vi "colorScatterRandomGenerator.vi"(8 "error in":errorcluster, 11 "Control in":refnum<vi>) -> (0 "error out":errorcluster)   [LabVIEW 2023]
uses:
  <vilib>/Math Plots/3D Math Plots/3D Scatter/3D Scatter XCtrl/3D Scatter.xctl
  <vilib>/Math Plots/3D Math Plots/3D Plot/3D Plot/Typedef/Color Ramp Cluster.ctl
  <vilib>/Math Plots/3D Math Plots/3D Plot/3D Plot/Typedef/Sprite Type.ctl
  <vilib>/Math Plots/3D Math Plots/3D Plot/3D Plot/3D Plot.lvclass
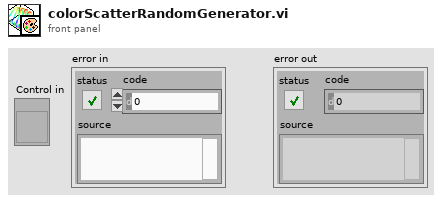
[diagram p1: front panel]
types:
  T1 = typedef "3D Plot.lvclass/Sprite Type.ctl" = enum16{"None", "Empty Square", "Solid Square", "Empty Diamond", "Solid Diamond", "Empty Circle", "Solid Circle", "Asterisk", "Bold X", "Wireframe Sphere", "Solid Sphere", "Wireframe Cube", "Solid Cube"}
  T2 = enum16{"None", "Shaded", "Color spectrum", "Grey scale", "Custom"}
  T3 = typedef "3D Plot.lvclass/Color Ramp Cluster.ctl" = cluster{"Color Ramp Style":enum16{"None", "Shaded", "Color spectrum", "Grey scale", "Custom"}, "Color Ramp Array":u32[], "Color Ramp Index":i32[], "Interpolate?":bool, "Logarithm?":bool}
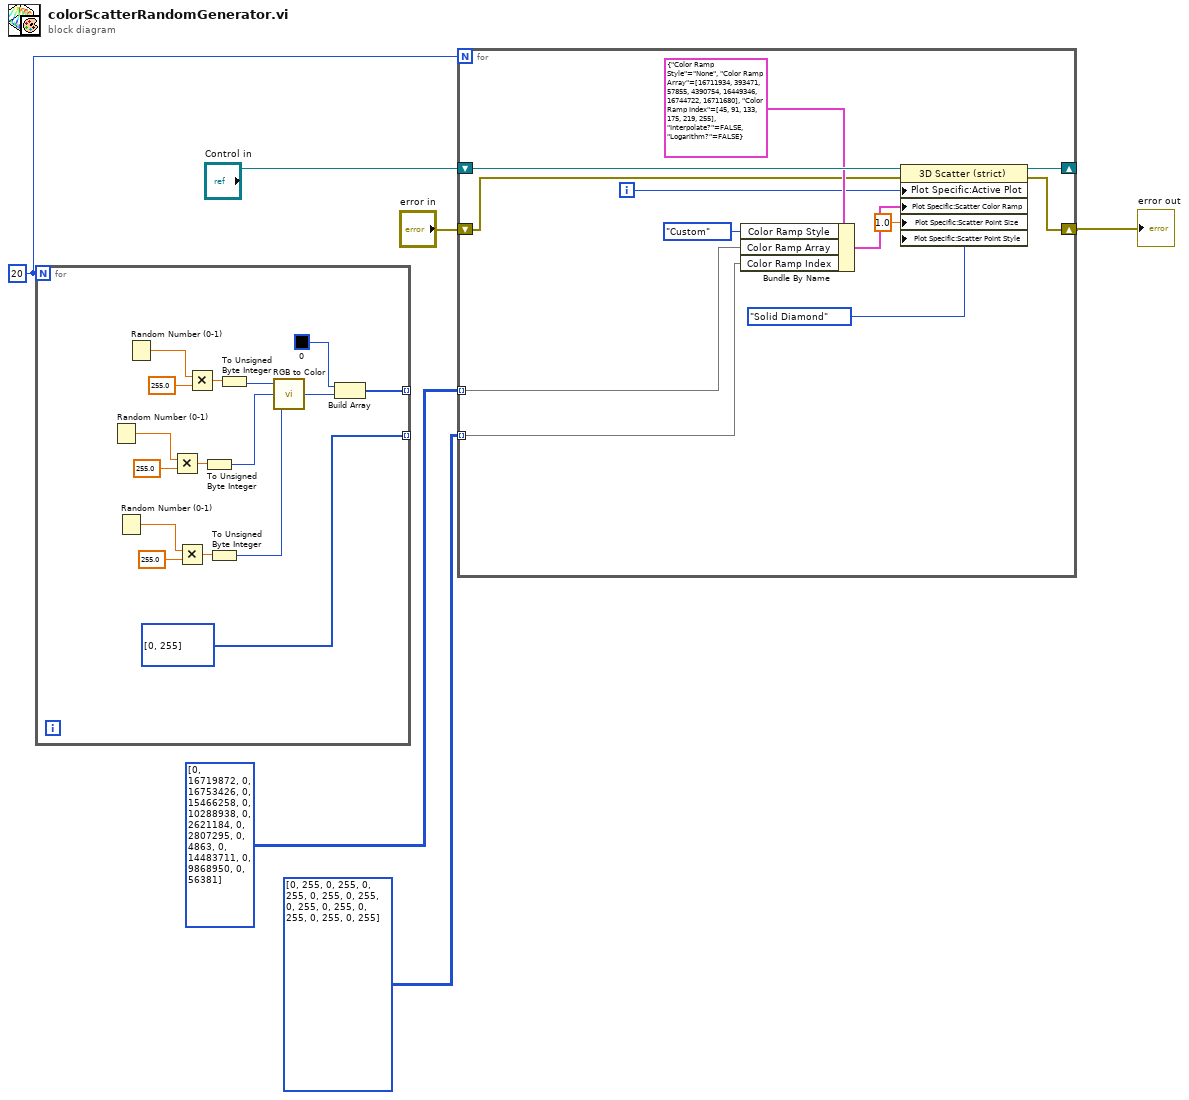
[diagram p0: block diagram]
diagram:
  w5 = 20
  n1 = for {
    N: w5 -> [_]
    tunnel: [w8] -> _ mode=indexing
    tunnel: [i32[] [0, 255] ("Color Ramp Index")] -> _ mode=indexing
    n2 = Random Number (0-1)() -> (number: 0 to 1=w18:dbl)
    n3 = Random Number (0-1)() -> (number: 0 to 1=w17:dbl)
    n4 = Random Number (0-1)() -> (number: 0 to 1=w22:dbl)
    n5 = Multiply(x=w18, y=255.0) -> (x*y=w19:dbl)
    n6 = Multiply(x=w17, y=255.0) -> (x*y=w16:dbl)
    n7 = Multiply(x=w22, y=255.0) -> (x*y=w21:dbl)
    n8 = To Unsigned Byte Integer(number=w19) -> (unsigned 8bit integer=w15:u8)
    n9 = To Unsigned Byte Integer(number=w16) -> (unsigned 8bit integer=w14:u8)
    n10 = To Unsigned Byte Integer(number=w21) -> (unsigned 8bit integer=w20:u8)
    n11 = call <vilib>:"RGB to Color.vi"("B"=w14, "G"=w15, "R"=w20) -> ("Color"=w13:u32)
    n12 = Build Array(u32 0 ("Color Box"), w13) -> (w8:u32[])
  }
  n13 = for {
    N: w5 -> [_]
    tunnel: u32[][] [[0, 16719872], [0, 16753426], [0, 15466258], [0, 10288938], [0, 2621184], [0, 2807295], [0, 4863], [0, 14483711], [0, 9868950], [0, 56381]] -> [w30] mode=indexing
    tunnel: i32[][] [[0, 255], [0, 255], [0, 255], [0, 255], [0, 255], [0, 255], [0, 255], [0, 255], [0, 255], [0, 255]] ("Color Ramp Index") -> [w29] mode=indexing
    shift-right: [w26] -> _
    shift-left: "Control in" -> [w34]
    shift-right: [w25] -> w4
    shift-left: "error in" -> [w24]
    i -> [w23]
    n14 = Bundle By Name(cluster=T3 {"Color Ramp Style"=enum."None", "Color Ramp Array"=[16711934, 393471, 57855, 4390754, 16449346, 16744722, 16711680], "Color Ramp Index"=[45, 91, 133, 175, 219, 255], "Interpolate?"=FALSE, "Logarithm?"=FALSE} ("Plot Specific:Scatter:Scatter Color Ramp"), "Color Ramp Style"=T2."Custom", "Color Ramp Array"=w30, "Color Ramp Index"=w29) -> (w32:T3)
    n15 = property class="3D Scatter (strict)"(reference=w34, error in=w24, "Plot Specific:Active Plot"=w23, "Plot Specific:Scatter Color Ramp"=w32, "Plot Specific:Scatter Point Size"=sgl 1.0 ("Plot Specific:Scatter:Scatter Point Size"), "Plot Specific:Scatter Point Style"=Sprite_Type."Solid Diamond" ("Plot Specific:Scatter:Scatter Point Style")) -> (reference out=w26:refnum<vi>, error out=w25:errorcluster)
  }
  "error out" <- w4
